vi "NI-RFSG_Configure RF.vi"(8 "error in":errorcluster, 9 "Level":dbl=-90.0 format="%.2f", 10 "Frequency (Hz)":dbl=100000000.0 format="%.2p", 11 "Handle In":variant) -> (0 "error out":errorcluster {"code" format="%.0x"}, 3 "Handle Out":variant)   [LabVIEW 2015]
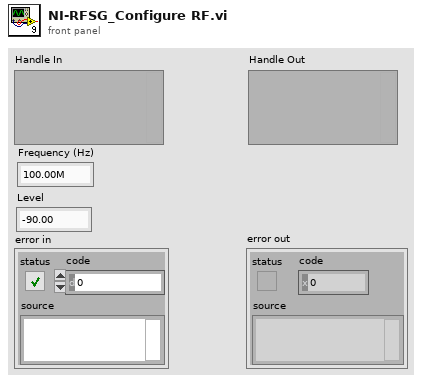
[diagram p1: front panel]
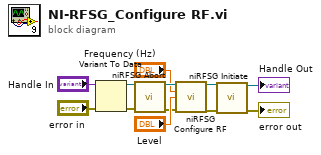
[diagram p0: block diagram]
diagram:
  n1 = Variant To Data(error in="error in", Variant="Handle In") -> (data=w10:refnum<k15>, error out=w9:errorcluster)  [unwired: 1 in]
  n2 = call <instrlib>:"niRFSG Abort.vi"("instrument handle"=w10, "error in"=w9) -> ("instrument handle out"=w8:refnum<k15>, "error out"=w5:errorcluster)  [unwired: 12 in]
  n3 = call <instrlib>:"niRFSG Configure RF.vi"("instrument handle"=w8, "frequency (Hz)"="Frequency (Hz)", "power level (dBm)"="Level", "error in"=w5) -> ("instrument handle out"=w4:refnum<k15>, "error out"=w3:errorcluster)  [unwired: 10 in]
  n4 = call <instrlib>:"niRFSG Initiate.vi"("instrument handle"=w4, "error in"=w3) -> ("instrument handle out"=→"Handle Out":refnum<k15>, "error out"=→"error out":errorcluster)  [unwired: 12 in]
